vi "Unflatten Name.vi"(8 "error in (no error)":errorcluster, 11 "Data String":string) -> (0 "error out":errorcluster, 2 "Rest of String":string, 3 "Name":string)   [LabVIEW 2015, in "Scripting.lvlib"]
uses:
  Scripting.lvlib
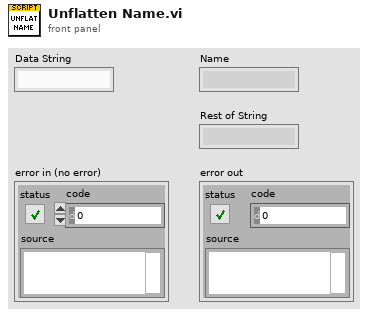
[diagram p1: front panel]
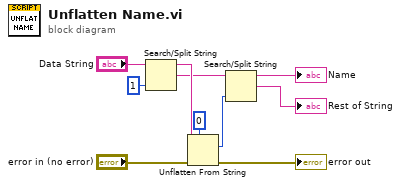
[diagram p0: block diagram]
diagram:
  n1 = Search/Split String(string="Data String", offset (0)=1) -> (substring before match=w9:string, match + rest of string=w5:string)  [unwired: 1 in, 1 out]
  n2 = Unflatten From String(type=u8 0, binary string=w9, error in (no error)="error in (no error)") -> (value=w10:u8, error out=→"error out":errorcluster)  [unwired: 2 in, 1 out]
  n3 = Search/Split String(string=w5, offset (0)=w10) -> (substring before match=→"Name":string, match + rest of string=→"Rest of String":string)  [unwired: 1 in, 1 out]
